vi "Score Display - Auto Scale Image (LV).vi"(1 "Picture Reference":refnum<vi>, 2 "path to image file":path) -> (0 "error out":errorcluster)   [LabVIEW 2013]
uses:
  <vilib>/Utility/miscctls.llb/LVBoundsTypeDef.ctl
  <vilib>/picture/picture.llb/imagedata.ctl
  Instance           4 45Saved   Score Display - Auto Scale Image (LV) .vi
panel:
  out "Draw Area Size":T1
  in  "Path to file that references image":path
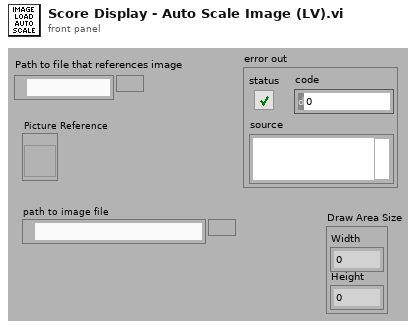
[diagram p1: front panel]
types:
  T1 = typedef "LVBoundsTypeDef.ctl" = cluster{"Width":u32, "Height":u32}
  T2 = typedef "imagedata.ctl" = cluster{"image type":i32, "image depth":i32, "image":u8[], "mask":u8[], "colors":u32[], "Rectangle":cluster{"left":i16, "top":i16, "right":i16, "bottom":i16}}
  T3 = cluster{"left":i16, "top":i16, "right":i16, "bottom":i16}
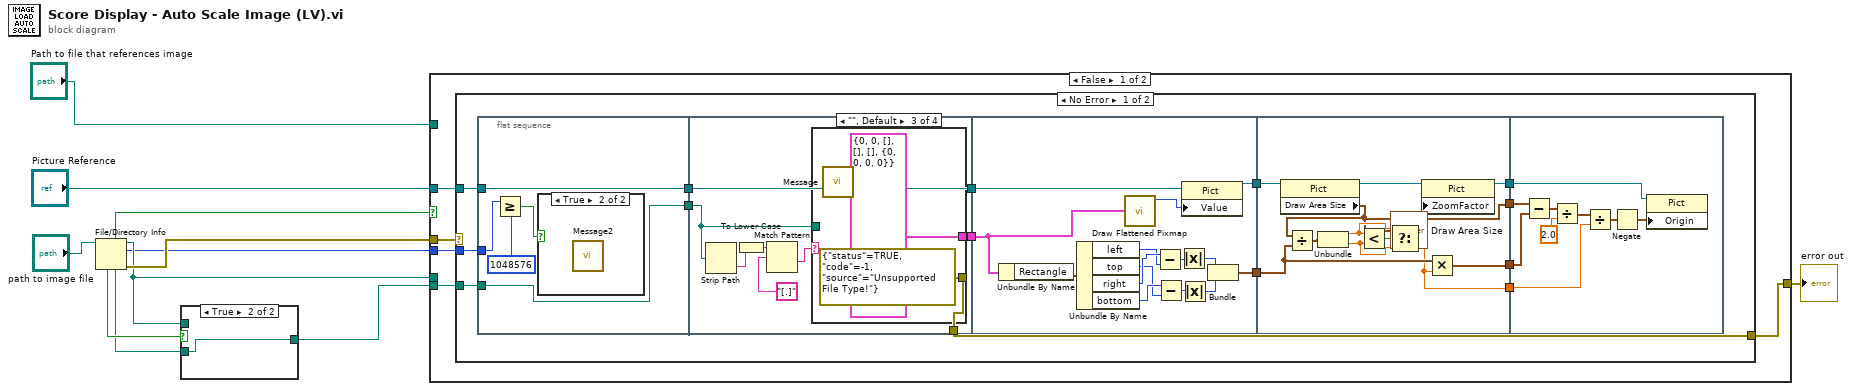
[diagram p0: block diagram]
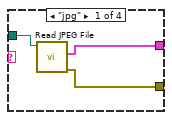
[diagram p3: hidden frame]
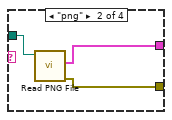
[diagram p4: hidden frame]
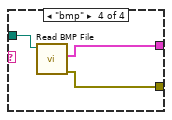
[diagram p5: hidden frame]
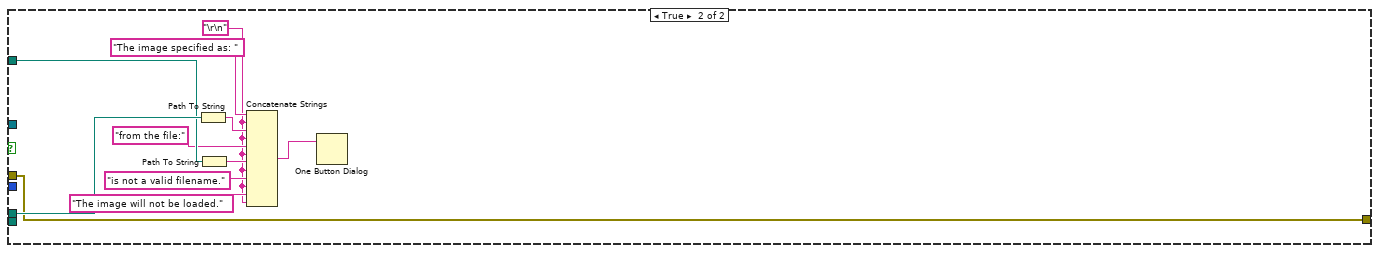
[diagram p7: hidden frame]
diagram:
  n1 = File/Directory Info(path="path to image file") -> (path out=w4:path, directory=w5:bool, size=w2:i64, error out=w7:errorcluster, resolved path=w8:path, shortcut=w9:bool)  [unwired: 1 in, 1 out]
  n2 = case shown="True" w9 {
    tunnel: w4 -> [w12 _]
    tunnel: w8 -> [_ w13]
    tunnel: [w12 w13] -> w6
    frame False {
    }
    frame True {
    }
  }
  n3 = case shown="False" w5 {
    tunnel: "Picture Reference" -> [w18 _]
    tunnel: w7 -> [w17 w91]
    tunnel: w6 -> [w16 _]
    tunnel: w4 -> [_ w101]
    tunnel: "Path to file that references image" -> [_ w100]
    tunnel: w2 -> [w15 _]
    tunnel: [w14 w91] -> w1
    frame False {
      n4 = case shown="No Error" w17 {
        selector: w17 -> [_ w90]
        tunnel: w18 -> [w22 _]
        tunnel: w16 -> [w21 _]
        tunnel: w15 -> [w20 _]
        tunnel: [w19 w90] -> w14
        frame No Error {
          n5 = flat-sequence {
            tunnel: w22 -> [w37]
            tunnel: [w33] -> w32
            tunnel: [w37] -> w31
            tunnel: w21 -> [w33]
            tunnel: w20 -> [w36]
            tunnel: [w45] -> w30
            tunnel: [w42] -> w29
            tunnel: w32 -> [w43]
            tunnel: w31 -> [w45]
            tunnel: [w38] -> w19
            tunnel: [w62] -> w28
            tunnel: [w59] -> w27
            tunnel: w30 -> [w61]
            tunnel: w29 -> [w58]
            tunnel: w28 -> [w76]
            tunnel: [w75] -> w26
            tunnel: [w70] -> w25
            tunnel: [w73] -> w24
            tunnel: w27 -> [w74]
            tunnel: [w71] -> w23
            tunnel: w26 -> [w88]
            tunnel: w25 -> [w89]
            tunnel: w24 -> [w84]
            tunnel: w23 -> [w81]
            frame #0 {
              n6 = Greater Or Equal?(x=w36, y=1048576) -> (x >= y?=w34:bool)
              n7 = case shown="True" w34 {
                frame False {
                }
                frame True {
                  n8 = call "Message2"() -> ()  [unwired: 3 in, 9 out]
                }
              }
            }
            frame #1 {
              n9 = Strip Path(path=w43) -> (name=w40:string)  [unwired: 1 out]
              n10 = To Lower Case(string=w40) -> (all lower case string=w39:string)
              n11 = Match Pattern(string=w39, regular expression="[.]") -> (after substring=w41:string)  [unwired: 4 out]
              n12 = case shown="\"\", Default" w41 {
                tunnel: w43 -> [w47 w51 _ w56]
                tunnel: [w48 w50 T2 {"image type"=0, "image depth"=0, "image"=[], "mask"=[], "colors"=[], "Rectangle"={"left"=0, "top"=0, "right"=0, "bottom"=0}} ("image data") w55] -> w42
                tunnel: [w46 w49 errorcluster {"status"=TRUE, "code"=-1, "source"="Unsupported File Type!"} ("error constant") w54] -> w38
                frame "jpg" {
                  n13 = call <vilib>:"Read JPEG File.vi"("path to JPEG file"=w47) -> ("error out"=w46:errorcluster, "image data"=w48:T2)  [unwired: 1 in, 8 out]
                }
                frame "png" {
                  n14 = call <vilib>:"Read PNG File.vi"("path to PNG file"=w51) -> ("error out"=w49:errorcluster, "image data"=w50:T2)  [unwired: 1 in, 8 out]
                }
                frame "", Default {
                  n15 = call "Message"() -> ()  [unwired: 3 in, 9 out]
                }
                frame "bmp" {
                  n16 = call <vilib>:"Read BMP File.vi"("path to BMP file"=w56) -> ("error out"=w54:errorcluster, "image data"=w55:T2)  [unwired: 1 in, 8 out]
                }
              }
            }
            frame #2 {
              n17 = Unbundle By Name(w58) -> ("Rectangle"=w57:T3)
              n18 = Unbundle By Name(w57) -> ("left"=w68:i16, "top"=w66:i16, "right"=w69:i16, "bottom"=w67:i16)
              n19 = call <vilib>:"Draw Flattened Pixmap.vi"("image data"=w58) -> ("new picture"=w60:picture)  [unwired: 1 in, 7 out]
              n20 = Subtract(x=w69, y=w68) -> (x-y=w64:i16)
              n21 = Subtract(x=w67, y=w66) -> (x-y=w65:i16)
              n22 = Absolute Value(x=w64) -> ()  [unwired: 1 out]
              n23 = Absolute Value(x=w65) -> (abs(x)=w63:i16)
              n24 = property class="Pict"(reference=w61, "Value"=w60) -> (reference out=w59:refnum<vi>)  [unwired: 1 in, 1 out]
              n25 = Bundle(w64, w63) -> (w62:cluster{i16, i16})  [unwired: 1 out]
            }
            frame #3 {
              n26 = property class="Pict"(reference=w74) -> (reference out=w72:refnum<vi>, "Draw Area Size"=w70:T1)  [unwired: 1 in, 1 out]
              "Draw Area Size" <- w70
              n27 = Divide(x=w70, y=w76) -> (x/y=w80:cluster{dbl, dbl})
              n28 = Unbundle(w80) -> (w78:dbl, w77:dbl)
              n29 = Less?(x=w78, y=w77) -> (x < y?=w79:bool)
              n30 = Select(t=w78, s=w79, f=w77) -> (s? t:f=w73:dbl)
              n31 = property class="Pict"(reference=w72, "ZoomFactor"=w73) -> (reference out=w71:refnum<vi>)  [unwired: 1 in, 1 out]
              n32 = Multiply(x=w76, y=w73) -> (x*y=w75:cluster{dbl, dbl})
            }
            frame #4 {
              n33 = Subtract(x=w89, y=w88) -> (x-y=w86:cluster{dbl, dbl})
              n34 = Divide(x=w86, y=2.0) -> (x/y=w85:cluster{dbl, dbl})
              n35 = Divide(x=w85, y=w84) -> (x/y=w83:cluster{dbl, dbl})
              n36 = Negate(x=w83) -> (-x=w82:cluster{dbl, dbl})
              n37 = property class="Pict"(reference=w81, "Origin"=w82) -> ()  [unwired: 1 in, 2 out]
            }
          }
        }
        frame Error {
        }
      }
    }
    frame True {
      w92 = "\r\n"
      n38 = Path To String(path=w101) -> (string=w98:string)
      n39 = Path To String(path=w100) -> (string=w96:string)
      n40 = Concatenate Strings("The image specified as: ", w92, w98, w92, "from the file:", w92, w96, w92, "is not a valid filename.", w92, "The image will not be loaded.", w92) -> (w94:string)
      n41 = One Button Dialog(message=w94) -> ()  [unwired: 2 out]
    }
  }
  "error out" <- w1
